vi "Write VISA resource name.vi"(8 "error in (no error)":errorcluster, 10 "VISA resource name":refnum<visa-resource-name>="SR_PS350", 11 "Power Supply in":refnum<class "Power Supply.lvclass">) -> (0 "error out":errorcluster, 3 "Power Supply out":refnum<class "Power Supply.lvclass">)   [LabVIEW 2011, in "Power Supply.lvclass"]
uses:
  Power Supply.lvclass
  Power Supply.lvclass/Power Supply.ctl
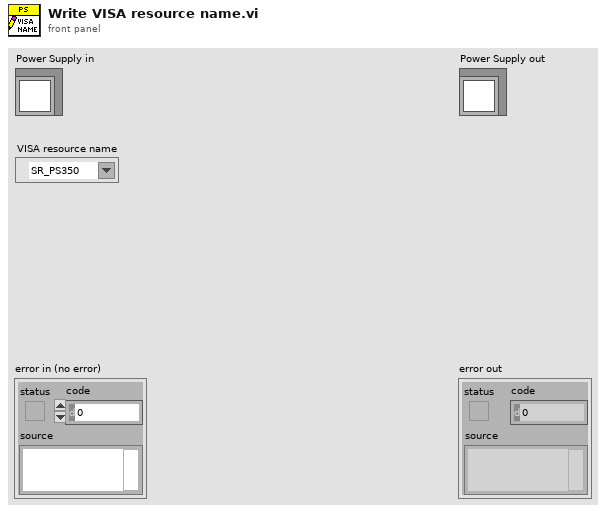
[diagram p1: front panel]
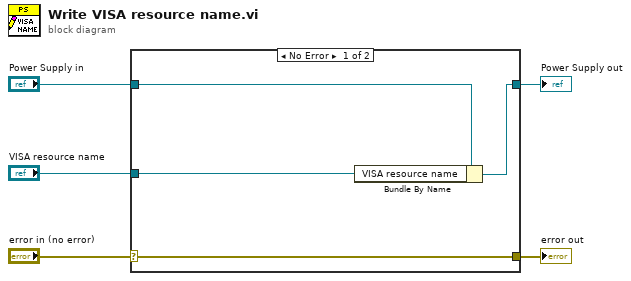
[diagram p0: block diagram]
diagram:
  n1 = case shown="No Error" "error in (no error)" {
    selector: "error in (no error)" -> [w9 w10]
    tunnel: [w9 w10] -> w4
    tunnel: [w7 w11] -> w2
    tunnel: "Power Supply in" -> [w8 w11]
    tunnel: "VISA resource name" -> [w6 _]
    frame No Error {
      n2 = Bundle By Name(cluster=w8, "VISA resource name"=w6) -> (w7:refnum<class "Power Supply.lvclass">)
    }
    frame Error {
    }
  }
  "error out" <- w4
  "Power Supply out" <- w2
